vi "Emballage_BDD_continuer_Cmd_sans_melange_des_lots.vi"(6 "Continuer?":bool, 8 "indice lot IN":i32, 9 "Numero carton IN":i32, 10 "Nombre de pièce \nds dernier carton IN":i32, 11 "Tableau lots OUT":string[][](array[string])=[["0801", "13"], ["0802", "7"], ["0803", "11"]]) -> (0 "indice lot OUT":i32, 1 "Numero carton OUT":i32, 2 "Nombre de pièce ds dernier carton OUT":i32, 3 "Tableau lots OUT 2":string[][](array[string])=[["0801", "13"], ["0802", "7"], ["0803", "11"]])   [LabVIEW 2020]
panel:
  out "lots precedent":string
  out "lots à faire":string
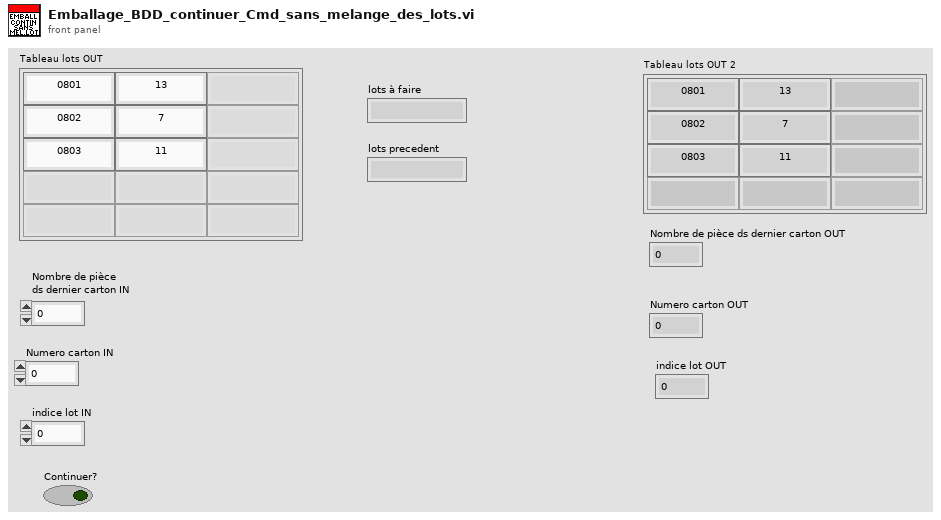
[diagram p1: front panel]
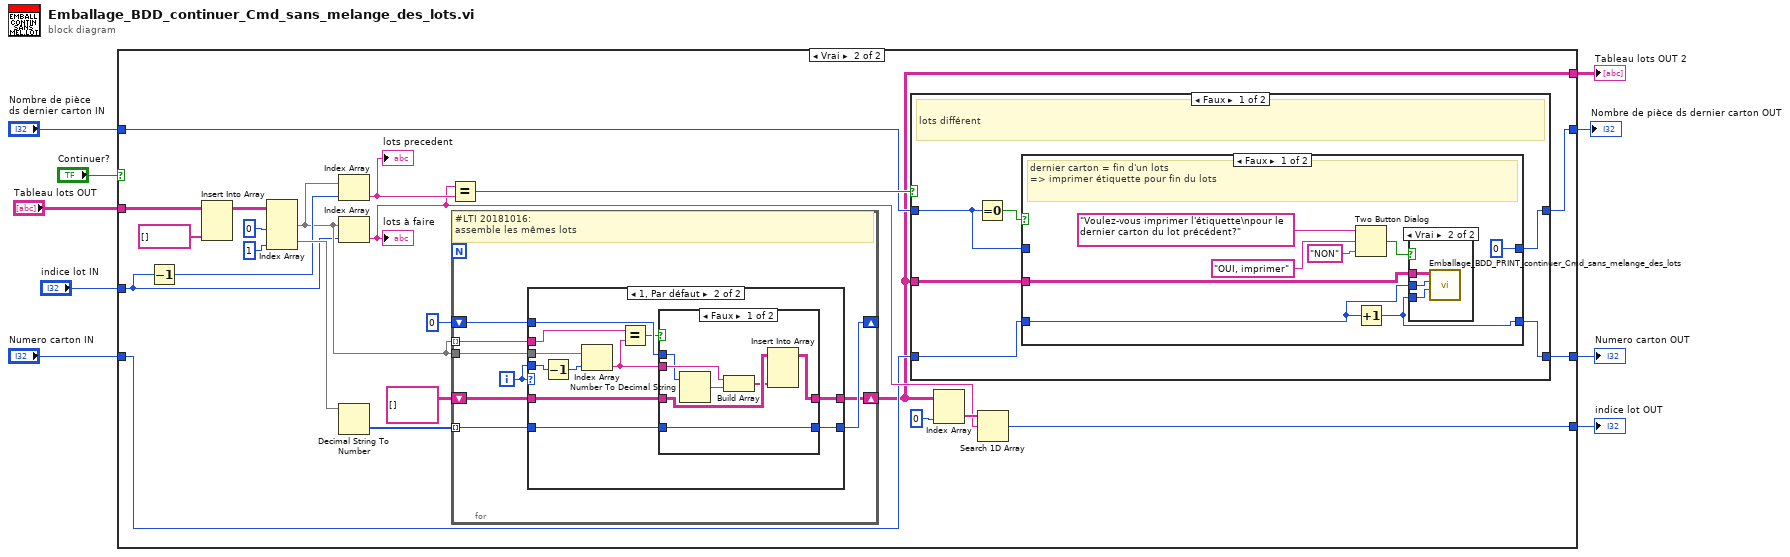
[diagram p0: block diagram]
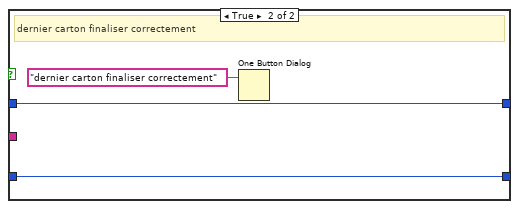
[diagram p4: hidden frame]
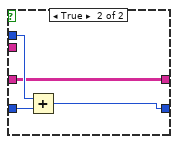
[diagram p7: hidden frame]
diagram:
  n1 = case shown="Vrai" "Continuer?" {
    tunnel: [w12 w21] -> w8
    tunnel: [w11 w20] -> w7
    tunnel: [w10 w19] -> w6
    tunnel: [w13 w14] -> w5
    tunnel: "Tableau lots OUT" -> [w13 w18]
    tunnel: "indice lot IN" -> [w12 w17]
    tunnel: "Nombre de pièce \nds dernier carton IN" -> [w11 w16]
    tunnel: "Numero carton IN" -> [w10 w15]
    frame False {
    }
    frame True {
      n2 = Decrement(x=w17) -> (x-1=w28:i32)
      n3 = Insert Into Array(array=w18, new element=string[] [] ("nouvel élément/sous-tableau")) -> (w30:string[][])  [unwired: 2 in]
      n4 = Index Array(array=w30, index (col) #1=0 ("indice désactivé (col)"), index (col) #2=1 ("indice (col)")) -> (element #1=w27:string[], element #2=w34:string[])  [unwired: 2 in]
      n5 = Index Array(array=w27, index=w28) -> (element=w26:string)
      "lots precedent" <- w26
      n6 = Index Array(array=w27, index=w17) -> (element=w22:string)
      "lots à faire" <- w22
      n7 = Decimal String To Number(string=w34) -> (number=w29:i32[])  [unwired: 2 in, 1 out]
      n8 = Equal?(x=w22, y=w26) -> (x = y?=w25:bool)
      n9 = for {
        tunnel: w27 -> [w61] mode=indexing
        tunnel: w27 -> [w66]
        tunnel: w29 -> [w63] mode=indexing
        shift-right: [w62] -> _
        shift-left: 0 -> [w64]
        shift-right: [w59] -> w14
        shift-left: string[][] [] -> [w60]
        i -> [w65]
        # "#LTI 20181016:\nassemble les mêmes lots"
        n10 = case shown="1, Par défaut" w65 {
          tunnel: w66 -> [_ w79]
          tunnel: w65 -> [_ w78]
          tunnel: w61 -> [_ w77]
          tunnel: w64 -> [_ w75]
          tunnel: w63 -> [w68 w74]
          tunnel: [w68 w72] -> w62
          tunnel: w60 -> [w67 w71]
          tunnel: [w67 w69] -> w59
          frame 0 {
          }
          frame 1, Default {
            n11 = Decrement(x=w78) -> (x-1=w76:i32)
            n12 = Index Array(array=w79, index=w76) -> (element=w70:string)
            n13 = Equal?(x=w77, y=w70) -> (x = y?=w73:bool)
            n14 = case shown="Faux" w73 {
              tunnel: w75 -> [w80 w90]
              tunnel: w74 -> [w86 w89]
              tunnel: [w86 w88] -> w72
              tunnel: w71 -> [w85 w87]
              tunnel: w70 -> [w83 _]
              tunnel: [w82 w87] -> w69
              frame False {
                n15 = Number To Decimal String(number=w80) -> (decimal integer string=w81:string)  [unwired: 1 in]
                n16 = Build Array(w83, w81) -> (w84:string[])
                n17 = Insert Into Array(array=w85, new element=w84) -> (w82:string[][])  [unwired: 2 in]
              }
              frame True {
                n18 = Add(x=w90, y=w89) -> (x+y=w88:i32)
              }
            }
          }
        }
      }
      n19 = case shown="Faux" w25 {
        tunnel: w16 -> [w41 w58]
        tunnel: [w40 w58] -> w20
        tunnel: w15 -> [w38 w57]
        tunnel: [w39 w57] -> w19
        tunnel: w14 -> [w37 _]
        frame False {
          # "lots différent"
          n20 = Equal To 0?(x=w41) -> (x = 0?=w42:bool)
          n21 = case shown="Faux" w42 {
            tunnel: [0 ("Nombre de pièce ds dernier carton") w55] -> w40
            tunnel: w38 -> [w47 w54]
            tunnel: [w46 w54] -> w39
            tunnel: w41 -> [_ w55]
            tunnel: w37 -> [w48 _]
            frame False {
              # "dernier carton = fin d'un lots\n=> imprimer étiquette pour fin du lots"
              n22 = Two Button Dialog(message="Voulez-vous imprimer l'étiquette\npour le dernier carton du lot précédent?", 1:"NON" ("Nom du bouton F (\"Annuler\")"), 2:"OUI, imprimer" ("Nom du bouton V (\"OK\")")) -> (T button?=w45:bool)
              n23 = Increment(x=w47) -> (x+1=w46:i32)
              n24 = case shown="Vrai" w45 {
                tunnel: w48 -> [_ w53]
                tunnel: w47 -> [_ w52]
                tunnel: w46 -> [_ w51]
                frame False {
                }
                frame True {
                  n25 = call "Emballage_BDD_PRINT_continuer_Cmd_sans_melange_des_lots.vi"("Carton prochain Numéro"=w51, "N° carton"=w52, "Tableau \nlots OUT"=w53) -> ()  [unwired: 8 in, 1 out]
                }
              }
            }
            frame True {
              # "dernier carton finaliser correctement"
              n26 = One Button Dialog(message="dernier carton finaliser correctement") -> ()  [unwired: 1 in, 1 out]
            }
          }
        }
        frame True {
          # "même lots\n=> rien faire"
        }
      }
      n27 = Index Array(array=w14, index (col)=0 ("indice désactivé (col)")) -> (element=w23:string[])  [unwired: 1 in]
      n28 = Search 1D Array(1D array=w23, element=w22) -> (index of element=w21:i32)  [unwired: 1 in]
    }
  }
  "indice lot OUT" <- w8
  "Nombre de pièce ds dernier carton OUT" <- w7
  "Numero carton OUT" <- w6
  "Tableau lots OUT 2" <- w5
